vi "Lab Panel V5.22.1.vi"() -> ()   [LabVIEW 2013] (continued)
                n1762 = property on="SELECT LAB01-1" class="RadioBtnsControl (strict)"("DisabledEnum"=w3329) -> ()  [unwired: 2 in, 2 out]
                n1763 = property on="SELECT LAB01-2" class="RadioBtnsControl (strict)"("DisabledEnum"=w3328) -> ()  [unwired: 2 in, 2 out]
                n1764 = Not(x=w3338) -> (.not. x?=w3339:bool)
                n1765 = property on="RESULT LAB01-1" class="Bool (strict)"("Visible"=w3339) -> ()  [unwired: 2 in, 2 out]
                n1766 = Not(x=w3333) -> (.not. x?=w3337:bool)
                n1767 = Not(x=w3332) -> (.not. x?=w3336:bool)
                n1768 = Not(x=w3330) -> (.not. x?=w3335:bool)
                n1769 = property on="RESULT LAB01-2" class="Bool (strict)"("Visible"=w3337) -> ()  [unwired: 2 in, 2 out]
                n1770 = Not(x=w3331) -> (.not. x?=w3334:bool)
                n1771 = property on="RESULT LAB02-1" class="Bool (strict)"("Visible"=w3336) -> ()  [unwired: 2 in, 2 out]
                n1772 = property on="RESULT LAB02-2" class="Bool (strict)"("Visible"=w3335) -> ()  [unwired: 2 in, 2 out]
                n1773 = property on="RESULT LAB03-1" class="Bool (strict)"("Visible"=w3334) -> ()  [unwired: 2 in, 2 out]
                n1774 = property on="SET LAB01-1" class="Clust (strict)"("DisabledEnum"=w3329) -> ()  [unwired: 2 in, 2 out]
                n1775 = property on="SET LAB01-2" class="Clust (strict)"("DisabledEnum"=w3328) -> ()  [unwired: 2 in, 2 out]
                n1776 = property on="SET LAB02-1" class="Clust (strict)"("DisabledEnum"=w3327) -> ()  [unwired: 2 in, 2 out]
                n1777 = property on="SET LAB02-2" class="Clust (strict)"("DisabledEnum"=w3326) -> ()  [unwired: 2 in, 2 out]
                n1778 = property on="SET LAB03-1" class="Clust (strict)"("DisabledEnum"=w3325) -> ()  [unwired: 2 in, 2 out]
                n1779 = property on="O/I  LAB01-1" class="Bool (strict)"("DisabledEnum"=w3329) -> ()  [unwired: 2 in, 2 out]
                n1780 = property on="O/I  LAB01-2" class="Bool (strict)"("DisabledEnum"=w3328) -> ()  [unwired: 2 in, 2 out]
                n1781 = property on="O/I  LAB02-1" class="Bool (strict)"("DisabledEnum"=w3327) -> ()  [unwired: 2 in, 2 out]
                n1782 = property on="O/I  LAB02-2" class="Bool (strict)"("DisabledEnum"=w3326) -> ()  [unwired: 2 in, 2 out]
                n1783 = property on="O/I  LAB03-1" class="Bool (strict)"("DisabledEnum"=w3325) -> ()  [unwired: 2 in, 2 out]
              }
              frame #1 {
                n1784 = Select(t=2, s=w3359, f=0) -> (s? t:f=w3350:i32)
                n1785 = Select(t=2, s=w3358, f=0) -> (s? t:f=w3351:i32)
                n1786 = Select(t=2, s=w3355, f=0) -> (s? t:f=w3354:i32)
                n1787 = Select(t=2, s=w3356, f=0) -> (s? t:f=w3353:i32)
                n1788 = Select(t=2, s=w3357, f=0) -> (s? t:f=w3352:i32)
                n1789 = property on="SELECT LAB05-2" class="RadioBtnsControl (strict)"("DisabledEnum"=w3350) -> ()  [unwired: 2 in, 2 out]
                n1790 = property on="SELECT LAB05-1" class="RadioBtnsControl (strict)"("DisabledEnum"=w3351) -> ()  [unwired: 2 in, 2 out]
                n1791 = property on="SELECT LAB03-2" class="RadioBtnsControl (strict)"("DisabledEnum"=w3354) -> ()  [unwired: 2 in, 2 out]
                n1792 = property on="SELECT LAB04-1" class="RadioBtnsControl (strict)"("DisabledEnum"=w3353) -> ()  [unwired: 2 in, 2 out]
                n1793 = property on="SELECT LAB04-2" class="RadioBtnsControl (strict)"("DisabledEnum"=w3352) -> ()  [unwired: 2 in, 2 out]
                n1794 = property on="SET LAB05-2" class="Clust (strict)"("DisabledEnum"=w3350) -> ()  [unwired: 2 in, 2 out]
                n1795 = property on="SET LAB05-1" class="Clust (strict)"("DisabledEnum"=w3351) -> ()  [unwired: 2 in, 2 out]
                n1796 = property on="SET LAB03-2" class="Clust (strict)"("DisabledEnum"=w3354) -> ()  [unwired: 2 in, 2 out]
                n1797 = property on="SET LAB04-1" class="Clust (strict)"("DisabledEnum"=w3353) -> ()  [unwired: 2 in, 2 out]
                n1798 = property on="SET LAB04-2" class="Clust (strict)"("DisabledEnum"=w3352) -> ()  [unwired: 2 in, 2 out]
                n1799 = property on="O/I  LAB05-2" class="Bool (strict)"("DisabledEnum"=w3350) -> ()  [unwired: 2 in, 2 out]
                n1800 = property on="O/I  LAB05-1" class="Bool (strict)"("DisabledEnum"=w3351) -> ()  [unwired: 2 in, 2 out]
                n1801 = property on="O/I  LAB04-1" class="Bool (strict)"("DisabledEnum"=w3353) -> ()  [unwired: 2 in, 2 out]
                n1802 = property on="O/I  LAB04-2" class="Bool (strict)"("DisabledEnum"=w3352) -> ()  [unwired: 2 in, 2 out]
                n1803 = property on="O/I  LAB03-2" class="Bool (strict)"("DisabledEnum"=w3354) -> ()  [unwired: 2 in, 2 out]
                n1804 = Not(x=w3359) -> (.not. x?=w3360:bool)
                n1805 = Not(x=w3358) -> (.not. x?=w3361:bool)
                n1806 = Not(x=w3357) -> (.not. x?=w3362:bool)
                n1807 = property on="RESULT LAB05-2" class="Bool (strict)"("Visible"=w3360) -> ()  [unwired: 2 in, 2 out]
                n1808 = property on="RESULT LAB05-1" class="Bool (strict)"("Visible"=w3361) -> ()  [unwired: 2 in, 2 out]
                n1809 = Not(x=w3356) -> (.not. x?=w3363:bool)
                n1810 = property on="RESULT LAB04-2" class="Bool (strict)"("Visible"=w3362) -> ()  [unwired: 2 in, 2 out]
                n1811 = Not(x=w3355) -> (.not. x?=w3364:bool)
                n1812 = property on="RESULT LAB04-1" class="Bool (strict)"("Visible"=w3363) -> ()  [unwired: 2 in, 2 out]
                n1813 = property on="RESULT LAB03-2" class="Bool (strict)"("Visible"=w3364) -> ()  [unwired: 2 in, 2 out]
              }
              frame #2 {
                # "disable calibrate if any test running"
                n1814 = Or(x=w3387, y=w3386) -> (x .or. y?=w3380:bool)
                n1815 = Or(x=w3389, y=w3388) -> (x .or. y?=w3382:bool)
                n1816 = Or(x=w3393, y=w3392) -> (x .or. y?=w3384:bool)
                n1817 = Or(x=w3391, y=w3390) -> (x .or. y?=w3383:bool)
                n1818 = Or(x=w3395, y=w3394) -> (x .or. y?=w3385:bool)
                n1819 = Or(x=w3383, y=w3382) -> (x .or. y?=w3381:bool)
                n1820 = Or(x=w3385, y=w3384) -> (x .or. y?=w3379:bool)
                n1821 = Or(x=w3381, y=w3380) -> (x .or. y?=w3378:bool)
                n1822 = Or(x=w3379, y=w3378) -> (x .or. y?=w3377:bool)
                n1823 = case shown="False" w3377 {
                  tunnel: [0 2] -> w3376
                  frame False {
                  }
                  frame True {
                  }
                }
                n1824 = property on="JIG TEST" class="Clust (strict)"("DisabledEnum"=w3376) -> ()  [unwired: 2 in, 2 out]
                n1825 = property on="Network Directory" class="Path"("DisabledEnum"=w3376) -> ()  [unwired: 2 in, 2 out]
                n1826 = property on="MAIL SETTINGS" class="Clust (strict)"("DisabledEnum"=w3376) -> ()  [unwired: 2 in, 2 out]
                n1827 = property on="SET (cal)" class="Bool (strict)"("DisabledEnum"=w3376) -> ()  [unwired: 2 in, 2 out]
                n1828 = property on="ADMIN" class="Bool (strict)"("DisabledEnum"=0) -> ()  [unwired: 2 in, 2 out]
              }
            }
          }
          frame #8 {
            # "drive jigs"
            n1829 = stacked-sequence {
              frame #0 {
                # "jig on"
                n1830 = local read "jig cycle"() -> (w3403:dbl)
                n1831 = property on="JIG TEST" class="Clust (strict)"() -> ("DisabledEnum"=w3400:T16)  [unwired: 2 in, 2 out]
                n1832 = Equal?(x=w3400, y=2) -> (x = y?=w3399:bool)
                n1833 = Equal?(x=w3403, y=0) -> (x = y?=w3401:bool)
                n1834 = And(x=w3401, y=w3399) -> (x .and. y?=w3398:bool)
                n1835 = case shown="True" w3398 {
                  frame False {
                  }
                  frame True {
                    n1836 = local read "run lab01-1"() -> (w3414:bool)
                    n1837 = local read "run lab01-2"() -> (w3413:bool)
                    n1838 = local read "run lab02-1"() -> (w3412:bool)
                    n1839 = local read "run lab02-2"() -> (w3411:bool)
                    n1840 = local read "run lab03-1"() -> (w3410:bool)
                    n1841 = local read "run lab03-2"() -> (w3409:bool)
                    n1842 = local read "run lab04-1"() -> (w3408:bool)
                    n1843 = local read "run lab04-2"() -> (w3407:bool)
                    n1844 = local read "run lab05-1"() -> (w3406:bool)
                    n1845 = local read "run lab05-2"() -> (w3405:bool)
                    n1846 = local write "JIG LAB03-2"(w3409) -> ()
                    n1847 = local write "JIG LAB01-1"(w3414) -> ()
                    n1848 = local write "JIG LAB01-2"(w3413) -> ()
                    n1849 = local write "JIG LAB02-1"(w3412) -> ()
                    n1850 = local write "JIG LAB02-2"(w3411) -> ()
                    n1851 = local write "JIG LAB03-1"(w3410) -> ()
                    n1852 = local write "JIG LAB04-1"(w3408) -> ()
                    n1853 = local write "JIG LAB04-2"(w3407) -> ()
                    n1854 = local write "JIG LAB05-1"(w3406) -> ()
                    n1855 = local write "JIG LAB05-2"(w3405) -> ()
                  }
                }
              }
              frame #1 {
                # "jig off"
                n1856 = local read "jig cycle"() -> (w3421:dbl)
                n1857 = local read "on loops"() -> (w3420:dbl)
                n1858 = property on="JIG TEST" class="Clust (strict)"() -> ("DisabledEnum"=w3419:T16)  [unwired: 2 in, 2 out]
                n1859 = Equal?(x=w3419, y=2) -> (x = y?=w3417:bool)
                n1860 = Equal?(x=w3421, y=w3420) -> (x = y?=w3416:bool)
                n1861 = And(x=w3416, y=w3417) -> (x .and. y?=w3415:bool)
                n1862 = case shown="True" w3415 {
                  frame False {
                  }
                  frame True {
                    w3472 = FALSE
                    w3473 = TRUE
                    w3471 = 2
                    n1863 = local read "SELECT LAB05-2"() -> (w3462:T3)
                    n1864 = local read "SELECT LAB04-2"() -> (w3464:T3)
                    n1865 = local read "SELECT LAB04-1"() -> (w3465:T3)
                    n1866 = local read "SELECT LAB05-1"() -> (w3463:T3)
                    n1867 = local read "SELECT LAB03-2"() -> (w3466:T3)
                    n1868 = local read "SELECT LAB02-1"() -> (w3469:T3)
                    n1869 = local read "SELECT LAB03-1"() -> (w3467:T3)
                    n1870 = local read "SELECT LAB02-2"() -> (w3468:T3)
                    n1871 = local read "SELECT LAB01-2"() -> (w3470:T3)
                    n1872 = local read "run lab05-1"() -> (w3432:bool)
                    n1873 = local read "run lab05-2"() -> (w3431:bool)
                    n1874 = local read "SELECT LAB01-1"() -> (w3474:T3)
                    n1875 = local read "run lab04-2"() -> (w3433:bool)
                    n1876 = local read "run lab04-1"() -> (w3434:bool)
                    n1877 = local read "run lab01-1"() -> (w3450:bool)
                    n1878 = local read "run lab01-2"() -> (w3439:bool)
                    n1879 = local read "run lab03-2"() -> (w3435:bool)
                    n1880 = local read "run lab03-1"() -> (w3436:bool)
                    n1881 = local read "run lab02-1"() -> (w3438:bool)
                    n1882 = local read "run lab02-2"() -> (w3437:bool)
                    n1883 = Equal?(x=w3471, y=w3467) -> (x = y?=w3445:bool)
                    n1884 = Equal?(x=w3471, y=w3466) -> (x = y?=w3444:bool)
                    n1885 = Equal?(x=w3471, y=w3465) -> (x = y?=w3443:bool)
                    n1886 = Equal?(x=w3471, y=w3464) -> (x = y?=w3442:bool)
                    n1887 = Equal?(x=w3471, y=w3463) -> (x = y?=w3441:bool)
                    n1888 = Equal?(x=w3471, y=w3462) -> (x = y?=w3440:bool)
                    n1889 = Equal?(x=w3471, y=w3474) -> (x = y?=w3451:bool)
                    n1890 = Equal?(x=w3471, y=w3469) -> (x = y?=w3447:bool)
                    n1891 = Equal?(x=w3471, y=w3468) -> (x = y?=w3446:bool)
                    n1892 = Equal?(x=w3471, y=w3470) -> (x = y?=w3448:bool)
                    n1893 = And(x=w3442, y=w3433) -> (x .and. y?=w3424:bool)
                    n1894 = And(x=w3445, y=w3436) -> (x .and. y?=w3427:bool)
                    n1895 = And(x=w3443, y=w3434) -> (x .and. y?=w3425:bool)
                    n1896 = And(x=w3440, y=w3431) -> (x .and. y?=w3422:bool)
                    n1897 = And(x=w3446, y=w3437) -> (x .and. y?=w3428:bool)
                    n1898 = And(x=w3444, y=w3435) -> (x .and. y?=w3426:bool)
                    n1899 = And(x=w3441, y=w3432) -> (x .and. y?=w3423:bool)
                    n1900 = And(x=w3448, y=w3439) -> (x .and. y?=w3430:bool)
                    n1901 = And(x=w3451, y=w3450) -> (x .and. y?=w3449:bool)
                    n1902 = And(x=w3447, y=w3438) -> (x .and. y?=w3429:bool)
                    n1903 = Select(t=w3473, s=w3449, f=w3472) -> (s? t:f=w3452:bool)
                    n1904 = Select(t=w3473, s=w3430, f=w3472) -> (s? t:f=w3453:bool)
                    n1905 = Select(t=w3473, s=w3429, f=w3472) -> (s? t:f=w3454:bool)
                    n1906 = Select(t=w3473, s=w3428, f=w3472) -> (s? t:f=w3455:bool)
                    n1907 = Select(t=w3473, s=w3427, f=w3472) -> (s? t:f=w3456:bool)
                    n1908 = Select(t=w3473, s=w3426, f=w3472) -> (s? t:f=w3457:bool)
                    n1909 = Select(t=w3473, s=w3425, f=w3472) -> (s? t:f=w3458:bool)
                    n1910 = Select(t=w3473, s=w3424, f=w3472) -> (s? t:f=w3459:bool)
                    n1911 = Select(t=w3473, s=w3423, f=w3472) -> (s? t:f=w3460:bool)
                    n1912 = Select(t=w3473, s=w3422, f=w3472) -> (s? t:f=w3461:bool)
                    n1913 = local write "JIG LAB03-2"(w3457) -> ()
                    n1914 = local write "JIG LAB02-1"(w3454) -> ()
                    n1915 = local write "JIG LAB02-2"(w3455) -> ()
                    n1916 = local write "JIG LAB01-2"(w3453) -> ()
                    n1917 = local write "JIG LAB03-1"(w3456) -> ()
                    n1918 = local write "JIG LAB01-1"(w3452) -> ()
                    n1919 = local write "JIG LAB05-2"(w3461) -> ()
                    n1920 = local write "JIG LAB04-1"(w3458) -> ()
                    n1921 = local write "JIG LAB05-1"(w3460) -> ()
                    n1922 = local write "JIG LAB04-2"(w3459) -> ()
                  }
                }
              }
            }
          }
          frame #9 {
            # "enable  jig test output if no test busy"
            n1923 = property on="JIG TEST" class="Clust (strict)"() -> ("DisabledEnum"=w3477:T16)  [unwired: 2 in, 2 out]
            n1924 = Equal?(x=w3477, y=0) -> (x = y?=w3475:bool)
            n1925 = case shown="True" w3475 {
              frame False {
              }
              frame True {
                n1926 = local read "JIG TEST"() -> (w3488:T10)
                n1927 = Unbundle(w3488) -> ("LAB01-1"=w3487:bool, "LAB01-2"=w3486:bool, "LAB02-1"=w3485:bool, "LAB02-2"=w3484:bool, "LAB03-1"=w3483:bool, "LAB03-2"=w3482:bool, "LAB04-1"=w3481:bool, "LAB04-2"=w3480:bool, "LAB05-1"=w3479:bool, "LAB05-2"=w3478:bool)
                n1928 = local write "JIG LAB05-1"(w3479) -> ()
                n1929 = local write "JIG LAB05-2"(w3478) -> ()
                n1930 = local write "JIG LAB04-1"(w3481) -> ()
                n1931 = local write "JIG LAB04-2"(w3480) -> ()
                n1932 = local write "JIG LAB03-2"(w3482) -> ()
                n1933 = local write "JIG LAB01-1"(w3487) -> ()
                n1934 = local write "JIG LAB02-1"(w3485) -> ()
                n1935 = local write "JIG LAB03-1"(w3483) -> ()
                n1936 = local write "JIG LAB01-2"(w3486) -> ()
                n1937 = local write "JIG LAB02-2"(w3484) -> ()
              }
            }
          }
          frame #10 {
            # "Drive digital output and reset USB and temperature network if required."
            n1938 = global read "Global display 3.vi" "cycle O/F"() -> (w3498:bool)
            n1939 = local read "O/I  LAB05-2"() -> (w3491:bool)
            n1940 = local read "O/I  LAB05-1"() -> (w3493:bool)
            n1941 = local read "JIG LAB05-2"() -> (w3490:bool)
            n1942 = local read "O/I  LAB04-2"() -> (w3495:bool)
            n1943 = local read "JIG LAB05-1"() -> (w3492:bool)
            n1944 = local read "JIG LAB04-2"() -> (w3494:bool)
            n1945 = local read "O/I  LAB03-1"() -> (w3509:bool)
            n1946 = local read "O/I  LAB04-1"() -> (w3505:bool)
            n1947 = local read "O/I  LAB02-1"() -> (w3513:bool)
            n1948 = local read "O/I  LAB02-2"() -> (w3511:bool)
            n1949 = local read "O/I  LAB03-2"() -> (w3507:bool)
            n1950 = local read "JIG LAB04-1"() -> (w3504:bool)
            n1951 = local read "JIG LAB03-2"() -> (w3506:bool)
            n1952 = local read "O/I  LAB01-2"() -> (w3515:bool)
            n1953 = local read "JIG LAB02-1"() -> (w3512:bool)
            n1954 = local read "JIG LAB02-2"() -> (w3510:bool)
            n1955 = local read "JIG LAB03-1"() -> (w3508:bool)
            n1956 = local read "O/I  LAB01-1"() -> (w3517:bool)
            n1957 = local read "JIG LAB01-2"() -> (w3514:bool)
            n1958 = local read "JIG LAB01-1"() -> (w3516:bool)
            n1959 = case shown="False" w3498 {
              tunnel: [w3622 FALSE] -> w3497
              frame False {
                n1960 = local read "Analog error"() -> (w3624:bool)
                n1961 = local read "Reset Measuring"() -> (w3623:bool)
                n1962 = local read "Error Temp"() -> (w3621:bool)
                n1963 = Or(x=w3623, y=w3624) -> (x .or. y?=w3620:bool)
                n1964 = Or(x=w3620, y=w3621) -> (x .or. y?=w3622:bool)
              }
              frame True {
              }
            }
            n1965 = Build Array(w3510, w3509, w3508, w3507, w3506, w3505, w3504) -> (w3502:bool[])
            n1966 = Build Array(w3517, w3516, w3515, w3514, w3513, w3512, w3511) -> (w3503:bool[])
            n1967 = Build Array(w3495, w3494, w3493, w3492, w3491, w3490, FALSE) -> (w3501:bool[])
            n1968 = Not(x=w3498) -> (.not. x?=w3499:bool)
            n1969 = local read "Simulate"() -> (w3500:bool)
            n1970 = And(x=w3499, y=w3497) -> (x .and. y?=w3496:bool)
            n1971 = stacked-sequence {
              tunnel: w3503 -> [w3521 w3527]
              tunnel: w3502 -> [w3520 w3526]
              tunnel: w3501 -> [w3519 w3525]
              tunnel: w3500 -> [w3518 w3528]
              tunnel: w3496 -> [_ w3529]
              frame #0 {
                # "drive outputs for normal use"
                n1972 = case shown="False" w3518 {
                  tunnel: w3521 -> [w3524 _]
                  tunnel: w3520 -> [w3523 _]
                  tunnel: w3519 -> [w3522 _]
                  frame False {
                    n1973 = call "sub vi - Drive Relays All v6.vi"("Array #2"=w3522, "Array #1"=w3523, "Array #0"=w3524) -> ()  [unwired: 8 in, 1 out]
                  }
                  frame True {
                  }
                }
              }
              frame #1 {
                # "USB  reset routine"
                n1974 = case shown="True" w3529 {
                  tunnel: w3528 -> [_ w3533]
                  tunnel: w3527 -> [_ w3532]
                  tunnel: w3526 -> [_ w3531]
                  tunnel: w3525 -> [_ w3530]
                  frame False {
                  }
                  frame True {
                    n1975 = stacked-sequence {
                      seq-local: [w3535 _ _ _ _] -> [_ w3541 _ _ _]
                      tunnel: w3533 -> [_ w3545 _ _ _]
                      tunnel: w3532 -> [_ w3544 _ _ _]
                      tunnel: w3531 -> [_ w3543 _ _ _]
                      tunnel: w3530 -> [_ w3542 _ _ _]
                      frame #0 {
                        n1976 = case shown="False" "Auto Reset" {
                          tunnel: [w3538 FALSE] -> w3536
                          frame False {
                            n1977 = Two Button Dialog(message="System reset") -> (T button?=w3538:bool)  [unwired: 2 in]
                          }
                          frame True {
                          }
                        }
                        n1978 = disable-structure shown="Disabled" {
                          frame Disabled {
                            n1979 = local write "Tab Control 2"(5) -> ()
                          }
                          frame Enabled {
                          }
                        }
                        n1980 = Or(x="Auto Reset", y=w3536) -> (x .or. y?=w3535:bool)
                      }
                      frame #1 {
                        n1981 = case shown="True" w3541 {
                          tunnel: w3545 -> [_ w3551]
                          tunnel: w3544 -> [_ w3550]
                          tunnel: w3543 -> [_ w3549]
                          tunnel: w3542 -> [_ w3548]
                          frame False {
                          }
                          frame True {
                            n1982 = stacked-sequence {
                              tunnel: w3551 -> [_ w3569 _]
                              tunnel: bool[] [] -> [w3554 w3568 w3578]
                              tunnel: w3550 -> [_ _ w3577]
                              tunnel: w3549 -> [w3553 _ w3576]
                              tunnel: w3548 -> [w3552 _ w3575]
                              tunnel: 3000 -> [w3555 _ w3574]
                              frame #0 {
                                # "switch off test stations for system reset"
                                n1983 = stacked-sequence {
                                tunnel: w3555 -> [w3559 w3563 w3565]
                                tunnel: w3554 -> [w3558 w3562 w3566]
                                tunnel: w3553 -> [w3557 _ _]
                                tunnel: w3552 -> [w3556 w3561 _]
                                frame #0 {
                                # "drive 1st 7 inputs"
                                n1984 = call "sub vi - Drive Relays All v6.vi"("Array #2"=w3556, "Array #1"=w3557, "Array #0"=w3558) -> ()  [unwired: 8 in, 1 out]
                                n1985 = call "Message Display V1.vi"("Message"="Delay off LAB 01-1 to 02-1", "Delay mS"=w3559) -> ()  [unwired: 10 in]
                                }
                                frame #1 {
                                # "drive 2nd 7 inputs"
                                n1986 = call "sub vi - Drive Relays All v6.vi"("Array #2"=w3561, "Array #1"=w3562, "Array #0"=w3562) -> ()  [unwired: 8 in, 1 out]
                                n1987 = call "Message Display V1.vi"("Message"="Delay off LAB 02-2 to 04-1", "Delay mS"=w3563) -> ()  [unwired: 10 in]
                                }
                                frame #2 {
                                # "drive 3rd 7 inputs"
                                n1988 = call "sub vi - Drive Relays All v6.vi"("Array #2"=w3566, "Array #1"=w3566, "Array #0"=w3566) -> ()  [unwired: 8 in, 1 out]
                                n1989 = call "Message Display V1.vi"("Message"="Delay off LAB 04-2 to 05-2", "Delay mS"=w3565) -> ()  [unwired: 10 in]
                                }
                                }
                              }
                              frame #1 {
                                # "reset all usb modules"
                                n1990 = stacked-sequence {
                                tunnel: w3569 -> [_ w3573]
                                tunnel: w3568 -> [w3571 _]
                                frame #0 {
                                n1991 = call "sub vi - Drive Relays All v6.vi"("Array #2"=bool[] [FALSE, FALSE, FALSE, FALSE, FALSE, FALSE, TRUE], "Array #1"=w3571, "Array #0"=w3571) -> ()  [unwired: 8 in, 1 out]
                                }
                                frame #1 {
                                n1992 = call "Reset Meas v 4.vi"("simulate"=w3573) -> ("Reset Error"=→"Reset Error":bool)  [unwired: 10 in]
                                }
                                }
                              }
                              frame #2 {
                                # "switch test stations back on after reset"
                                n1993 = stacked-sequence {
                                tunnel: w3578 -> [w3582 w3585 _]
                                tunnel: w3577 -> [w3581 w3587 w3592]
                                tunnel: w3574 -> [w3580 w3583 w3589]
                                tunnel: w3576 -> [_ w3586 w3591]
                                tunnel: w3575 -> [_ _ w3588]
                                frame #0 {
                                # "drive 1st 7 inputs"
                                n1994 = call "sub vi - Drive Relays All v6.vi"("Array #2"=w3582, "Array #1"=w3582, "Array #0"=w3581) -> ()  [unwired: 8 in, 1 out]
                                n1995 = call "Message Display V1.vi"("Message"="Delay on LAB 01-1 to 02-1", "Delay mS"=w3580) -> ()  [unwired: 10 in]
                                }
                                frame #1 {
                                # "drive 1st & 2nd outputs"
                                n1996 = call "sub vi - Drive Relays All v6.vi"("Array #2"=w3585, "Array #1"=w3586, "Array #0"=w3587) -> ()  [unwired: 8 in, 1 out]
                                n1997 = call "Message Display V1.vi"("Message"="Delay on LAB 02-2 to 04-1", "Delay mS"=w3583) -> ()  [unwired: 10 in]
                                }
                                frame #2 {
                                n1998 = call "sub vi - Drive Relays All v6.vi"("Array #2"=w3588, "Array #1"=w3591, "Array #0"=w3592) -> ()  [unwired: 8 in, 1 out]
                                n1999 = call "Message Display V1.vi"("Message"="Delay on LAB 04-2 to 05-2", "Delay mS"=w3589) -> ()  [unwired: 10 in]
                                }
                                }
                              }
                            }
                          }
                        }
                      }
                      frame #2 {
                        w3593 = 0
                        w3594 = FALSE
                        # "set all back to zero"
                        n2000 = local read "Total USB resets"() -> (w3596:dbl)
                        n2001 = local read "Resets Done"() -> (w3598:dbl)
                        n2002 = local write "Reset Measuring"(w3594) -> ()
                        n2003 = local write "Temp Er 04"(w3593) -> ()
                        n2004 = local write "Analog error"(w3594) -> ()
                        n2005 = local write "Temp Er 02"(w3593) -> ()
                        n2006 = local write "Temp Er 01"(w3593) -> ()
                        n2007 = local write "Temp Er 03"(w3593) -> ()
                        n2008 = local write "Temp Er 05"(w3593) -> ()
                        n2009 = local write "Er USB#2"(w3593) -> ()
                        n2010 = local write "Er USB#0"(w3593) -> ()
                        n2011 = local write "Er USB#1"(w3593) -> ()
                        n2012 = local write "Error Temp"(w3594) -> ()
                        n2013 = local write "Error USB #0"(w3594) -> ()
                        n2014 = local write "Error USB #1"(w3594) -> ()
                        n2015 = local write "Error USB #2"(w3594) -> ()
                        n2016 = Increment(x=w3596) -> (x+1=w3595:dbl)
                        n2017 = Increment(x=w3598) -> (x+1=→"Resets Done":dbl)
                        n2018 = local write "Total USB resets"(w3595) -> ()
                      }
                      frame #3 {
                        # "save reset value"
                        n2019 = String To Path(string="c:\\crabtree\\Set Up\\") -> (path=w3608:path)
                        n2020 = Build Path(base path=w3608, name or relative path="USB resets.bin") -> (appended path=w3601:path)
                        n2021 = Create Folder(path (use dialog)=w3608) -> (error out=w3600:errorcluster)  [unwired: 2 in, 2 out]
                        n2022 = local read "Total USB resets"() -> (w3599:dbl)
                        n2023 = call <vilib>:"Clear Errors.vi"("error in (no error)"=w3600) -> ()  [unwired: 6 in, 1 out]
                        n2024 = Open/Create/Replace File(file path (use dialog)=w3601, operation (0:open)=T17."replace or create") -> (refnum out=w3606:refnum<file>, error out=w3605:errorcluster)  [unwired: 4 in, 1 out]
                        n2025 = Write to Binary File(file (use dialog)=w3606, data=w3599, error in=w3605) -> (refnum out=w3604:refnum<file>, error out=w3603:errorcluster)  [unwired: 3 in, 1 out]
                        n2026 = Close File(refnum=w3604, error in=w3603) -> (error out=w3602:errorcluster)  [unwired: 1 out]
                        n2027 = local write "data file error"(w3602) -> ()
                      }
                      frame #4 {
                        # "mail reset value"
                        n2028 = local read "Total USB resets"() -> (w3616:dbl)
                        n2029 = local read "MAIL SETTINGS"() -> (w3612:T7)
                        n2030 = local read "Mail Test File To:"() -> (w3617:string)
                        n2031 = Number To Decimal String(number=w3616) -> (decimal integer string=w3614:string)  [unwired: 1 in]
                        n2032 = Unbundle(w3612) -> ("OUT SERVER ADDRESS"=w3619:string, "FROM ACCOUNT"=w3618:string)  [unwired: 5 out]
                        n2033 = Concatenate Strings("Total USB resets: ", w3614) -> (w3613:string)
                        n2034 = call "sub vi - send mail v5.vi"("TO:"=w3617, "subject"=w3613, "from"=w3618, "out going server"=w3619) -> ("error out"=w3611:errorcluster)  [unwired: 11 in]
                        n2035 = Bundle(cluster=w3612, "mail error"=w3611) -> ()  [unwired: 6 in, 1 out]
                      }
                    }
                  }
                }
              }
            }
          }
          frame #11 {
            # "get all analog values from USB devices"
            n2036 = local read "on loops"() -> (w3632:dbl)
            n2037 = local read "jig cycle"() -> (w3629:dbl)
            n2038 = Add(x=w3632, y=1) -> (x+y=w3630:dbl)
            n2039 = Equal?(x=w3629, y=1) -> (x = y?=w3626:bool)
            n2040 = Equal?(x=w3629, y=w3630) -> (x = y?=w3628:bool)
            n2041 = Or(x=w3626, y=w3628) -> (x .or. y?=w3627:bool)
            n2042 = global write "Global display 3.vi" "cycle O/F"(w3626) -> ()
            n2043 = case shown="True" w3627 {
              tunnel: w3626 -> [_ w3636]
              frame False {
              }
              frame True {
                n2044 = local read "Simulate"() -> (w3639:bool)
                n2045 = case shown="False" w3639 {
                  tunnel: [w3655 0.3 ("Analog loop time")] -> w3646
                  tunnel: [w3654 dynamicdata[] [] ("array GRAPH")] -> w3645
                  tunnel: [w3653 w3660] -> w3644
                  tunnel: [w3652 w3660] -> w3643
                  tunnel: [w3651 w3660] -> w3642
                  tunnel: [w3650 w3660] -> w3641
                  tunnel: [w3649 w3660] -> w3640
                  tunnel: w3636 -> [_ w3664]
                  tunnel: [w3648 "Ambient Volts"] -> w3635
                  tunnel: [w3647 bool[] []] -> w3634
                  frame False {
                    n2046 = call "sub vi - Read Analog All v9.3.vi"() -> ("Analog loop time"=w3655:dbl, "array GRAPH"=w3654:dynamicdata[], "LAB01"=w3653:T27, "LAB02"=w3652:T28, "LAB03"=w3651:T29, "LAB04"=w3650:T30, "deg C"=w3648:dbl, "USB Error"=w3647:bool[], "LAB05"=w3649:T31)  [unwired: 7 in]
                  }
                  frame True {
                    n2047 = local read "ON amps"() -> (w3658:dbl)
                    n2048 = local read "OFF amps"() -> (w3659:dbl)
                    n2049 = local read "VOLTS"() -> (w3662:dbl)
                    n2050 = local read "PF"() -> (w3661:dbl)
                    n2051 = Select(t=w3658, s=w3664, f=w3659) -> (s? t:f=w3663:dbl)
                    n2052 = Bundle("OFF amps"=w3663, "VOLTS"=w3662, "PF"=w3661, "OFF amps"=w3663, "VOLTS"=w3662, "PF"=w3661) -> (w3660:T32)  [unwired: 1 in]
                  }
                }
                n2053 = local read "Simulate"() -> (w3638:bool)
                n2054 = stacked-sequence {
                  seq-local: [w3669 _ _ _ _ _ _ _] -> [_ _ _ _ _ _ _ _]
                  seq-local: [w3668 _ _ _ _ _ _ _] -> [_ _ _ _ _ _ _ _]
                  seq-local: [w3667 _ _ _ _ _ _ _] -> [_ _ _ _ _ _ _ w3864]
                  tunnel: w3646 -> [_ w3722 _ _ _ _ _ _]
                  tunnel: w3645 -> [_ w3719 _ _ _ _ _ _]
                  tunnel: w3644 -> [_ _ w3749 _ _ _ _ _]
                  tunnel: w3643 -> [_ _ _ w3777 _ _ _ _]
                  tunnel: w3642 -> [_ _ _ _ w3805 _ _ _]
                  tunnel: w3641 -> [_ _ _ _ _ w3833 _ _]
                  tunnel: w3640 -> [_ _ _ _ _ _ w3861 _]
                  tunnel: w3638 -> [_ _ w3748 w3776 w3804 w3832 w3860 w3866]
                  tunnel: T14 {"1  (A) cal"=1.0, "1 (V) cal"=1.0, "1 (PF) cal"=1.0, "1 (TL) cal"=1.0, "1 (TN) cal"=1.0, "2 (A) cal"=1.0, "2 (V) cal"=1.0, "2 (PF) cal"=1.0, "2 (TL) cal"=1.0, "2 (TN) cal"=1.0} ("CAL LAB01") -> [_ _ w3747 w3775 w3803 w3831 w3859 _]
                  tunnel: w3635 -> [_ _ _ _ _ _ _ w3865]
                  tunnel: w3634 -> [w3672 _ _ _ _ _ _ _]
                  frame #0 {
                    n2055 = Index Array(array=w3672, index=2) -> (element=w3667:bool)
                    n2056 = Index Array(array=w3672, index=1) -> (element=w3668:bool)
                    n2057 = Index Array(array=w3672, index=0) -> (element=w3669:bool)
                    n2058 = local write "Error USB #2"(w3667) -> ()
                    n2059 = local write "Error USB #0"(w3669) -> ()
                    n2060 = local write "Error USB #1"(w3668) -> ()
                    n2061 = stacked-sequence {
                      tunnel: w3669 -> [w3676 _ _ _]
                      tunnel: w3668 -> [_ w3681 _ _]
                      tunnel: 0 -> [w3675 w3680 w3685 _]
                      tunnel: w3667 -> [_ _ w3686 _]
                      frame #0 {
                        n2062 = case shown="True" w3676 {
                          tunnel: w3675 -> [w3677 _]
                          frame False {
                            n2063 = local write "Er USB#0"(w3677) -> ()
                          }
                          frame True {
                            n2064 = local read "Er USB#0"() -> (w3679:dbl)
                            n2065 = Increment(x=w3679) -> (x+1=→"Er USB#0":dbl)
                          }
                        }
                      }
                      frame #1 {
                        n2066 = case shown="True" w3681 {
                          tunnel: w3680 -> [w3682 _]
                          frame False {
                            n2067 = local write "Er USB#1"(w3682) -> ()
                          }
                          frame True {
                            n2068 = local read "Er USB#1"() -> (w3684:dbl)
                            n2069 = Increment(x=w3684) -> (x+1=→"Er USB#1":dbl)
                          }
                        }
                      }
                      frame #2 {
                        n2070 = case shown="True" w3686 {
                          tunnel: w3685 -> [w3687 _]
                          frame False {
                            n2071 = local write "Er USB#2"(w3687) -> ()
                          }
                          frame True {
                            n2072 = local read "Er USB#2"() -> (w3689:dbl)
                            n2073 = Increment(x=w3689) -> (x+1=→"Er USB#2":dbl)
                          }
                        }
                      }
                      frame #3 {
                        w3695 = 5
                        n2074 = local read "Er USB#2"() -> (w3696:dbl)
                        n2075 = local read "Er USB#0"() -> (w3698:dbl)
                        n2076 = local read "Er USB#1"() -> (w3697:dbl)
                        n2077 = Greater Or Equal?(x=w3698, y=w3695) -> (x >= y?=w3693:bool)
                        n2078 = Greater Or Equal?(x=w3697, y=w3695) -> (x >= y?=w3692:bool)
                        n2079 = Greater Or Equal?(x=w3696, y=w3695) -> (x >= y?=w3691:bool)
                        n2080 = Or(x=w3693, y=w3692) -> (x .or. y?=w3694:bool)
                        n2081 = Or(x=w3694, y=w3691) -> (x .or. y?=→"Analog error":bool)
                      }
                    }
                  }
                  frame #1 {
                    # "display graph data on ADM page"
                    n2082 = local write "AI"(TRUE) -> ()
                    n2083 = global write "Global 1.vi" "RATE(Hz)"("RATE (Hz)") -> ()
                    n2084 = global write "Global 1.vi" "SAMPLES"("SAMPLES") -> ()
                    n2085 = Index Array(array=w3719, index=6) -> (element=→"LAB04-1 (GRAPH)":dynamicdata)
                    n2086 = Index Array(array=w3719, index=7) -> (element=→"LAB04-2 (GRAPH)":dynamicdata)
                    n2087 = Index Array(array=w3719, index=9) -> (element=→"LAB05-2 (GRAPH)":dynamicdata)
                    n2088 = Index Array(array=w3719, index=8) -> (element=→"LAB05-1 (GRAPH)":dynamicdata)
                    n2089 = Index Array(array=w3719, index=5) -> (element=→"LAB03-2 (GRAPH)":dynamicdata)
                    n2090 = Index Array(array=w3719, index=0) -> (element=→"LAB01-1 (GRAPH)":dynamicdata)
                    n2091 = Index Array(array=w3719, index=1) -> (element=→"LAB01-2 (GRAPH)":dynamicdata)
                    n2092 = Index Array(array=w3719, index=2) -> (element=→"LAB02-1 (GRAPH)":dynamicdata)
                    n2093 = Index Array(array=w3719, index=3) -> (element=→"LAB02-2 (GRAPH)":dynamicdata)
                    n2094 = Index Array(array=w3719, index=4) -> (element=→"LAB03-1 (GRAPH)":dynamicdata)
                    "AI loop time" <- w3722
                  }
                  frame #2 {
                    n2095 = case shown="False" w3748 {
                      tunnel: [w3750 w3751] -> w3746
                      tunnel: w3747 -> [_ w3751]
                      frame False {
                        n2096 = local read "CAL LAB01"() -> (w3750:T14)
                      }
                      frame True {
                      }
                    }
                    n2097 = Unbundle By Name(w3749) -> ("OFF amps"=w3745:dbl, "VOLTS"=w3744:dbl, "PF"=w3743:dbl, "OFF amps"=w3742:dbl, "VOLTS"=w3741:dbl, "PF"=w3740:dbl)
                    n2098 = Unbundle By Name(w3746) -> ("1  (A) cal"=w3739:dbl, "1 (V) cal"=w3738:dbl, "1 (PF) cal"=w3737:dbl, "2 (A) cal"=w3736:dbl, "2 (V) cal"=w3735:dbl, "2 (PF) cal"=w3734:dbl)  [unwired: 4 out]
                    n2099 = Multiply(x=w3745, y=w3739) -> (x*y=w3732:dbl)
                    n2100 = Multiply(x=w3744, y=w3738) -> (x*y=w3731:dbl)
                    n2101 = Multiply(x=w3743, y=w3737) -> (x*y=w3730:dbl)
                    n2102 = Multiply(x=w3742, y=w3736) -> (x*y=w3728:dbl)
                    n2103 = Multiply(x=w3741, y=w3735) -> (x*y=w3727:dbl)
                    n2104 = Multiply(x=w3740, y=w3734) -> (x*y=w3726:dbl)
                    n2105 = local read "SIG LAB01-1"() -> (w3733:T2)
                    n2106 = local read "SIG LAB01-2"() -> (w3729:T2)
                    n2107 = Bundle By Name(cluster=w3733, "AMPS"=w3732, "VOLTS"=w3731, "PF"=w3730) -> (w3725:T2)
                    n2108 = Bundle By Name(cluster=w3729, "AMPS"=w3728, "VOLTS"=w3727, "PF"=w3726) -> (w3724:T2)
                    n2109 = global write "Global display 1.vi" "SIG LAB01-2"(w3724) -> ()
                    n2110 = global write "Global display 1.vi" "SIG LAB01-1"(w3725) -> ()
                    n2111 = local write "SIG LAB01-2"(w3724) -> ()
                    n2112 = local write "SIG LAB01-1"(w3725) -> ()
                  }
                  frame #3 {
                    n2113 = Unbundle By Name(w3777) -> ("OFF amps"=w3773:dbl, "VOLTS"=w3772:dbl, "PF"=w3771:dbl, "OFF amps"=w3770:dbl, "VOLTS"=w3769:dbl, "PF"=w3768:dbl)
                    n2114 = case shown="True" w3776 {
                      tunnel: [w3778 w3779] -> w3774
                      tunnel: w3775 -> [_ w3779]
                      frame False {
                        n2115 = local read "CAL LAB02"() -> (w3778:T15)
                      }
                      frame True {
                      }
                    }
                    n2116 = Unbundle By Name(w3774) -> ("1  (A) cal"=w3767:dbl, "1 (V) cal"=w3766:dbl, "1 (PF) cal"=w3765:dbl, "2 (A) cal"=w3764:dbl, "2 (V) cal"=w3763:dbl, "2 (PF) cal"=w3762:dbl)  [unwired: 4 out]
                    n2117 = Multiply(x=w3773, y=w3767) -> (x*y=w3760:dbl)
                    n2118 = Multiply(x=w3772, y=w3766) -> (x*y=w3759:dbl)
                    n2119 = Multiply(x=w3771, y=w3765) -> (x*y=w3758:dbl)
                    n2120 = Multiply(x=w3770, y=w3764) -> (x*y=w3756:dbl)
                    n2121 = Multiply(x=w3769, y=w3763) -> (x*y=w3755:dbl)
                    n2122 = Multiply(x=w3768, y=w3762) -> (x*y=w3754:dbl)
                    n2123 = local read "SIG LAB02-1"() -> (w3761:T2)
                    n2124 = local read "SIG LAB02-2"() -> (w3757:T2)
                    n2125 = Bundle By Name(cluster=w3761, "AMPS"=w3760, "VOLTS"=w3759, "PF"=w3758) -> (w3753:T2)
                    n2126 = Bundle By Name(cluster=w3757, "AMPS"=w3756, "VOLTS"=w3755, "PF"=w3754) -> (w3752:T2)
                    n2127 = global write "Global display 1.vi" "SIG LAB02-1"(w3753) -> ()
                    n2128 = local write "SIG LAB02-2"(w3752) -> ()
                    n2129 = global write "Global display 1.vi" "SIG LAB02-2"(w3752) -> ()
                    n2130 = local write "SIG LAB02-1"(w3753) -> ()
                  }
                  frame #4 {
                    n2131 = Unbundle By Name(w3805) -> ("OFF amps"=w3801:dbl, "VOLTS"=w3800:dbl, "PF"=w3799:dbl, "OFF amps"=w3798:dbl, "VOLTS"=w3797:dbl, "PF"=w3796:dbl)
                    n2132 = case shown="True" w3804 {
                      tunnel: [w3806 w3807] -> w3802
                      tunnel: w3803 -> [_ w3807]
                      frame False {
                        n2133 = local read "CAL LAB03"() -> (w3806:T14)
                      }
                      frame True {
                      }
                    }
                    n2134 = Unbundle By Name(w3802) -> ("1  (A) cal"=w3795:dbl, "1 (V) cal"=w3794:dbl, "1 (PF) cal"=w3793:dbl, "2 (A) cal"=w3792:dbl, "2 (V) cal"=w3791:dbl, "2 (PF) cal"=w3790:dbl)  [unwired: 4 out]
                    n2135 = Multiply(x=w3801, y=w3795) -> (x*y=w3788:dbl)
                    n2136 = Multiply(x=w3800, y=w3794) -> (x*y=w3782:dbl)
                    n2137 = Multiply(x=w3799, y=w3793) -> (x*y=w3787:dbl)
                    n2138 = Multiply(x=w3798, y=w3792) -> (x*y=w3785:dbl)
                    n2139 = Multiply(x=w3797, y=w3791) -> (x*y=w3784:dbl)
                    n2140 = Multiply(x=w3796, y=w3790) -> (x*y=w3783:dbl)
                    n2141 = local read "SIG LAB03-1"() -> (w3789:T2)
                    n2142 = local read "SIG LAB03-2"() -> (w3786:T2)
                    n2143 = Bundle By Name(cluster=w3789, "AMPS"=w3788, "VOLTS"=w3782, "PF"=w3787) -> (w3781:T2)
                    n2144 = Bundle By Name(cluster=w3786, "AMPS"=w3785, "VOLTS"=w3784, "PF"=w3783) -> (w3780:T2)
                    n2145 = global write "Global display 1.vi" "SIG LAB03-1"(w3781) -> ()
                    n2146 = global write "Global display 1.vi" "SIG LAB03-2"(w3780) -> ()
                    n2147 = local write "SIG LAB03-2"(w3780) -> ()
                    n2148 = local write "SIG LAB03-1"(w3781) -> ()
                  }
                  frame #5 {
                    n2149 = case shown="False" w3832 {
                      tunnel: [w3834 w3835] -> w3830
                      tunnel: w3831 -> [_ w3835]
                      frame False {
                        n2150 = local read "CAL LAB04"() -> (w3834:T14)
                      }
                      frame True {
                      }
                    }
                    n2151 = Unbundle By Name(w3833) -> ("OFF amps"=w3829:dbl, "VOLTS"=w3828:dbl, "PF"=w3827:dbl, "OFF amps"=w3826:dbl, "VOLTS"=w3825:dbl, "PF"=w3824:dbl)
                    n2152 = Unbundle By Name(w3830) -> ("1  (A) cal"=w3823:dbl, "1 (V) cal"=w3822:dbl, "1 (PF) cal"=w3821:dbl, "2 (A) cal"=w3820:dbl, "2 (V) cal"=w3819:dbl, "2 (PF) cal"=w3818:dbl)  [unwired: 4 out]
                    n2153 = Multiply(x=w3829, y=w3823) -> (x*y=w3816:dbl)
                    n2154 = Multiply(x=w3828, y=w3822) -> (x*y=w3815:dbl)
                    n2155 = Multiply(x=w3827, y=w3821) -> (x*y=w3814:dbl)
                    n2156 = Multiply(x=w3826, y=w3820) -> (x*y=w3812:dbl)
                    n2157 = Multiply(x=w3825, y=w3819) -> (x*y=w3811:dbl)
                    n2158 = Multiply(x=w3824, y=w3818) -> (x*y=w3810:dbl)
                    n2159 = local read "SIG LAB04-1"() -> (w3817:T2)
                    n2160 = local read "SIG LAB04-2"() -> (w3813:T2)
                    n2161 = Bundle By Name(cluster=w3817, "AMPS"=w3816, "VOLTS"=w3815, "PF"=w3814) -> (w3809:T2)
                    n2162 = Bundle By Name(cluster=w3813, "AMPS"=w3812, "VOLTS"=w3811, "PF"=w3810) -> (w3808:T2)
                    n2163 = global write "Global display 1.vi" "SIG LAB04-2"(w3808) -> ()
                    n2164 = global write "Global display 1.vi" "SIG LAB04-1"(w3809) -> ()
                    n2165 = local write "SIG LAB04-2"(w3808) -> ()
                    n2166 = local write "SIG LAB04-1"(w3809) -> ()
                  }
                  frame #6 {
                    n2167 = Unbundle By Name(w3861) -> ("OFF amps"=w3857:dbl, "VOLTS"=w3838:dbl, "PF"=w3856:dbl, "OFF amps"=w3855:dbl, "VOLTS"=w3854:dbl, "PF"=w3853:dbl)
                    n2168 = case shown="False" w3860 {
                      tunnel: [w3862 w3863] -> w3858
                      tunnel: w3859 -> [_ w3863]
                      frame False {
                        n2169 = local read "CAL LAB05"() -> (w3862:T14)
                      }
                      frame True {
                      }
                    }
                    n2170 = Unbundle By Name(w3858) -> ("1  (A) cal"=w3852:dbl, "1 (V) cal"=w3851:dbl, "1 (PF) cal"=w3850:dbl, "2 (A) cal"=w3849:dbl, "2 (V) cal"=w3848:dbl, "2 (PF) cal"=w3847:dbl)  [unwired: 4 out]
                    n2171 = Multiply(x=w3857, y=w3852) -> (x*y=w3845:dbl)
                    n2172 = Multiply(x=w3838, y=w3851) -> (x*y=w3844:dbl)
                    n2173 = Multiply(x=w3856, y=w3850) -> (x*y=w3843:dbl)
                    n2174 = Multiply(x=w3855, y=w3849) -> (x*y=w3841:dbl)
                    n2175 = Multiply(x=w3854, y=w3848) -> (x*y=w3840:dbl)
                    n2176 = Multiply(x=w3853, y=w3847) -> (x*y=w3839:dbl)
                    n2177 = local read "SIG LAB05-1"() -> (w3846:T2)
                    n2178 = local read "SIG LAB05-2"() -> (w3842:T2)
                    n2179 = Bundle By Name(cluster=w3846, "AMPS"=w3845, "VOLTS"=w3844, "PF"=w3843) -> (w3837:T2)
                    n2180 = Bundle By Name(cluster=w3842, "AMPS"=w3841, "VOLTS"=w3840, "PF"=w3839) -> (w3836:T2)
                    n2181 = global write "Global display 1.vi" "SIG LAB05-1"(w3837) -> ()
                    n2182 = global write "Global display 1.vi" "SIG LAB05-2"(w3836) -> ()
                    n2183 = local write "SIG LAB05-2"(w3836) -> ()
                    n2184 = local write "SIG LAB05-1"(w3837) -> ()
                  }
                  frame #7 {
                    n2185 = case shown="False" w3864 {
                      tunnel: w3866 -> [w3868 _]
                      tunnel: w3865 -> [w3867 _]
                      frame False {
                        # "update ambient referance temperature"
                        n2186 = case shown="True" w3868 {
                          tunnel: [w3871 100.0] -> w3870
                          frame False {
                            n2187 = local read "TEMP REF cal"() -> (w3871:dbl)
                          }
                          frame True {
                          }
                        }
                        n2188 = local read "Panel #"() -> (w3869:dbl)
                        n2189 = case shown="1" w3869 {
                          tunnel: w3870 -> [_ w3877]
                          tunnel: w3867 -> [_ w3876]
                          frame 0, Default {
                          }
                          frame 1 {
                            n2190 = Multiply(x=w3877, y=w3876) -> (x*y=w3875:dbl)
                            n2191 = Subtract(x=w3875, y=272) -> (x-y=w3873:dbl)
                            "Amb Tp" <- w3873
                            n2192 = local write "Ref deg C"(w3873) -> ()
                          }
                        }
                        "deg C (volts)" <- w3867
                      }
                      frame True {
                      }
                    }
                  }
                }
              }
            }
          }
          frame #12 {
            # "save test data to file"
            n2193 = Get Date/Time In Seconds() -> (seconds since 1Jan1904=w3878:timestamp)
            "File Time Stamp" <- w3878
            n2194 = local read "on loops"() -> (w3897:dbl)
            n2195 = local read "jig cycle"() -> (w3894:dbl)
            n2196 = Format Date/Time String(time format string (%c)="%H:%M%:%S", seconds (now)=w3878) -> (date/time string=w3882:string)  [unwired: 1 in]
            n2197 = Add(x=w3897, y=2) -> (x+y=w3895:dbl)
            n2198 = Build Array(w3882) -> (w3881:string[])
            n2199 = Equal?(x=w3894, y=1) -> (x = y?=w3880:bool)
